vi "Simple Example.vi"() -> ()   [LabVIEW 2015, in "VC940.lvlib"]
uses:
  VC940.lvlib
panel:
  out "Connection":bool
  out "Display":string
  out "Iteration":i32
  in  "Port name":string="COM1"
  in  "Exit":bool
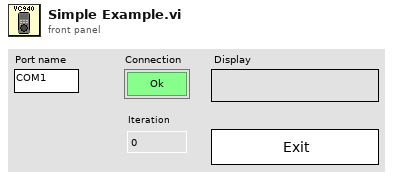
[diagram p1: front panel]
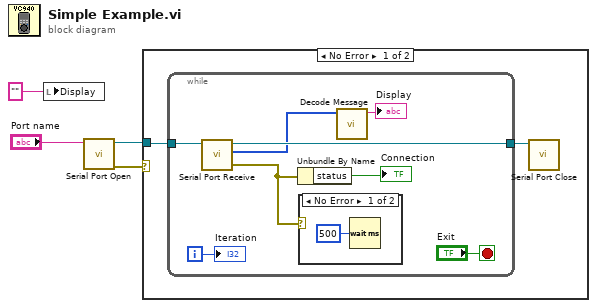
[diagram p0: block diagram]
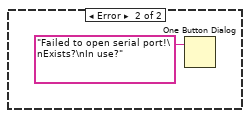
[diagram p3: hidden frame]
diagram:
  n1 = local write "Display"("" ("Data")) -> ()
  n2 = call "Serial Port Open.vi"("Port name (COM1)"="Port name") -> ("error out"=w1:errorcluster, "Port handle"=w3:refnum<k24>)  [unwired: 9 in]
  n3 = case shown="No Error" w1 {
    tunnel: w3 -> [w6 _]
    frame No Error {
      n4 = while {
        tunnel: w6 -> [w12]
        tunnel: [w11] -> w5
        i -> [w13]
        stop <- "Exit" stop-if-true
        n5 = call "Serial Port Receive.vi"("Port handle in"=w12) -> ("error out"=w9:errorcluster, "Message"=w7:u8[], "Port handle out"=w11:refnum<k24>)  [unwired: 8 in]
        n6 = Unbundle By Name(w9) -> ("status"=→"Connection":bool)
        n7 = case shown="No Error" w9 {
          frame No Error {
            n8 = Wait (ms)(milliseconds to wait=u32 500) -> ()  [unwired: 1 out]
          }
          frame Error {
          }
        }
        n9 = call "Decode Message.vi"("Message"=w7) -> ("Display string"=→"Display":string)  [unwired: 5 in, 5 out]
        "Iteration" <- w13
      }
      n10 = call "Serial Port Close.vi"("Port handle"=w5) -> ()  [unwired: 10 in, 1 out]
    }
    frame Error {
      n11 = One Button Dialog(message="Failed to open serial port!\nExists?\nIn use?") -> ()  [unwired: 1 in, 1 out]
    }
  }
